vi "Add Subentry.vi"(9 "OD Subentry":refnum<class "OD Subentry.lvclass">=refnum, 10 "Index":u8, 11 "OD Entry in":refnum<class "OD Entry.lvclass">) -> (3 "OD Entry out":refnum<class "OD Entry.lvclass">)   [LabVIEW 2024]
uses:
  OD Entry.lvclass/OD Entry.ctl
  OD Entry.lvclass
  OD Subentry/OD Subentry.lvclass
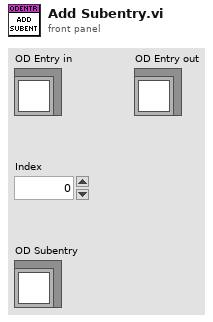
[diagram p1: front panel]
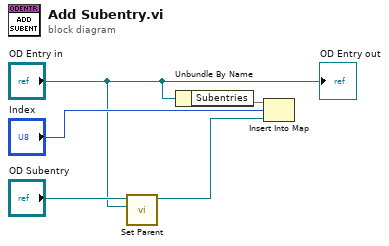
[diagram p0: block diagram]
diagram:
  n1 = call "Set Parent.vi"("EDS.lvlib:OD Entry.lvclass"="OD Entry in", "OD Subentry in"="OD Subentry") -> ("OD Subentry out"=w2:refnum<class "OD Subentry.lvclass">)  [unwired: 8 in, 1 out]
  n2 = Unbundle By Name("OD Entry in") -> ("Subentries"=w5)
  n3 = Insert Into Map(map in=w5, key="Index", value=w2) -> ()  [unwired: 3 out]
  "OD Entry out" <- "OD Entry in"
